vi "Delete Front Panel Objects.vi"(8 "error in (no error)":errorcluster, 11 "VI in":refnum<vi>) -> (0 "error out":errorcluster, 3 "VI out":refnum<vi>)   [LabVIEW 2018, in "Scripting.lvlib"]
uses:
  Scripting.lvlib
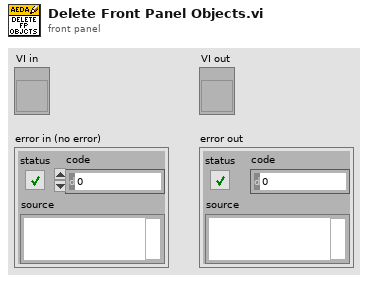
[diagram p1: front panel]
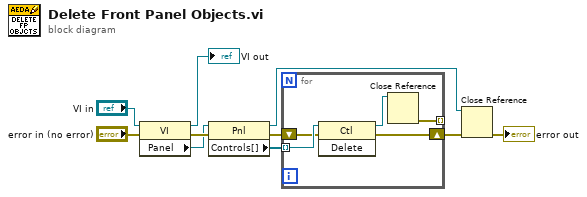
[diagram p0: block diagram]
diagram:
  n1 = property class="VI"(reference="VI in", error in="error in (no error)") -> (reference out=→"VI out":refnum<vi>, error out=w4:errorcluster, "Panel"=w2:refnum<vi>)
  n2 = property class="Pnl"(reference=w2, error in=w4) -> (reference out=w8:refnum<vi>, error out=w5:errorcluster, "Controls[]"=w6:refnum<vi>[])
  n3 = for {
    tunnel: w6 -> [w15] mode=indexing
    shift-right: [w12] -> w7
    shift-left: w5 -> [w14]
    tunnel: [w11] -> _ mode=indexing
    n4 = invoke class="Ctl" method="Delete"(reference=w15, error in=w14) -> (reference out=w13:refnum<vi>, error out=w12:errorcluster)  [unwired: 1 in, 1 out]
    n5 = Close Reference(reference=w13) -> (error out=w11:errorcluster)  [unwired: 1 in]
  }
  n6 = Close Reference(reference=w8, error in (no error)=w7) -> (error out=→"error out":errorcluster)
